vi "Register for DAQ Events.vi"(8 "error in (no error)":errorcluster, 11 "Get Daq Status in":refnum<class "Get Daq Status.lvclass">) -> (0 "error out":errorcluster, 1 "Process State":refnum<event-registration>, 2 "Daq events":refnum<event-registration>, 3 "Get Daq Status out":refnum<class "Get Daq Status.lvclass">)   [LabVIEW 2022 SP3, in "Get Daq Status.lvclass"]
uses:
  Get Daq Status.lvclass
  DAQ Data/AIDAQ Data.ctl
  DAQ Data/AI Daq Data.lvlib
  DAQ Data/Events.ctl
  DAQ Data/DAQ Data.lvclass
  XY Stage/Process Actor/Process Framework/Process State Data/Events.ctl
  XY Stage/Process Actor/Process Framework/Process State Data/Process State Data.lvclass
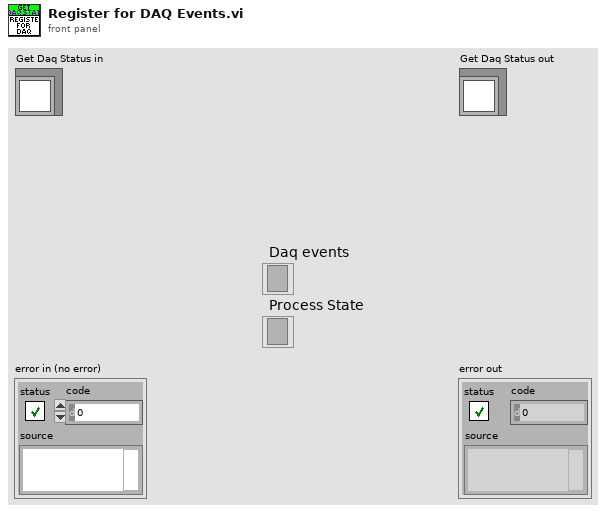
[diagram p1: front panel]
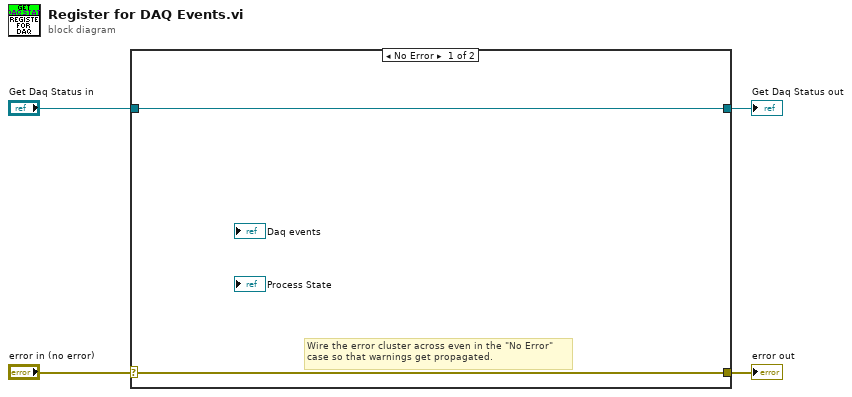
[diagram p0: block diagram]
diagram:
  n1 = case shown="No Error" "error in (no error)" {
    selector: "error in (no error)" -> [w5 w8]
    tunnel: [w5 w8] -> w3
    tunnel: [w6 w7] -> w1
    tunnel: "Get Daq Status in" -> [w6 w7]
    frame No Error {
      # "Wire the error cluster across even in the \"No Error\"\ncase so that warnings get propagated."
    }
    frame Error {
    }
  }
  "error out" <- w3
  "Get Daq Status out" <- w1
